vi "FRCts20_Backend_Error_To_Status.vi"(10 "error in (no error)":errorcluster, 11 "rows affected":i32) -> (2 "error out":errorcluster, 3 "String":string)   [LabVIEW 2014, in "FRCts20_Backend_Engine.lvlib"]
doc: "This Vi takes the number of rows affected by an sql command and the error returned, and converts that to a status message. That is, if there was no error and many rows were affected, we get a \"success\", while 0 rows affected or an error message is a failure."
uses:
  FRCts20_Backend_Engine.lvlib
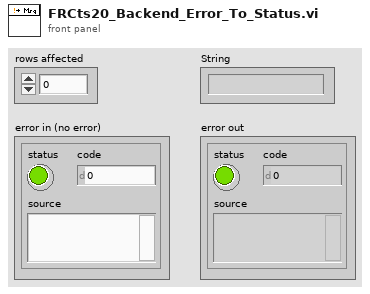
[diagram p1: front panel]
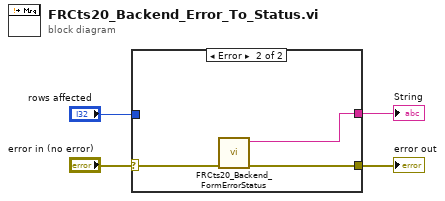
[diagram p0: block diagram]
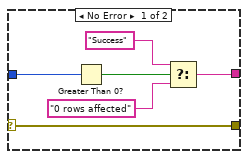
[diagram p2: hidden frame]
diagram:
  n1 = case shown="Error" "error in (no error)" {
    selector: "error in (no error)" -> [w10 w12]
    tunnel: [w10 w13] -> w2
    tunnel: [w7 w11] -> w4
    tunnel: "rows affected" -> [w9 _]
    frame No Error {
      n2 = Greater Than 0?(x=w9) -> (x > 0?=w8:bool)
      n3 = Select(t="Success", s=w8, f="0 rows affected") -> (s? t:f=w7:string)
    }
    frame Error {
      n4 = call "FRCts20_Backend_FormErrorStatus.vi"("error in (no error)"=w12) -> ("error out"=w13:errorcluster, "String"=w11:string)  [unwired: 9 in]
    }
  }
  "String" <- w4
  "error out" <- w2
